vi "Test Case Result Skipped Count.vi"(8 "error in (no error)":errorcluster, 11 "Test Test Case Result In":refnum<class "Test Case Result Test.lvclass">) -> (0 "error out":errorcluster, 3 "Test Test Case Result Out":refnum<class "Test Case Result Test.lvclass">)   [LabVIEW 2020, in "LUnit Tests.lvlib" / "Test Case Result Test.lvclass"]
uses:
  Test Case Result Test.lvclass
  C:/Program Files (x86)/National Instruments/LabVIEW 2020/vi.lib/Asteme/LUnit/Test Case.lvclass
  Test Dummys/Test Test Case/Test Test Case.lvclass
  C:/Users/anton/Documents/GitHub/LUnit/source/Framework/Test Case/LUnit Test Case.lvclass
  source/Framework/Result Classes/Test Case Result/Test Case Result.lvclass/Test Case Result.ctl
  source/Framework/Result Classes/Method Result/Method Result.lvclass/Method Result.ctl
  <vilib>/Asteme/LUnit/Test Case.lvclass/Test Case.ctl
  <vilib>/Asteme/LUnit/LUnit Assertion Result.lvclass/LUnit Assertion Result.ctl
  <vilib>/Asteme/LUnit/LUnit Test Case Result.lvclass/LUnit Test Case Result.ctl
  <vilib>/Asteme/LUnit/LUnit Method Result.lvclass/LUnit Method Result.ctl
  source/Framework/Result Classes/Test Case Result/Private/SubVIs/Count by Status.vi
  <vilib>/Asteme/LUnit/Palette/Pass.vi
  <vilib>/Asteme/LUnit/Palette/Fail.vi
  <vilib>/Asteme/LUnit/Variant to string.vi
  <vilib>/Asteme/LUnit/Set Assertion Type.vi
  source/Framework/Result Classes/Method Result/Public/Read Status.vi
  <vilib>/Asteme/LUnit/Add test result.vi
  <vilib>/Asteme/LUnit/LUnit Write Passed.vi
  <vilib>/Asteme/LUnit/LUnit Write Message.vi
  <vilib>/Asteme/LUnit/LUnit Write Description.vi
  <vilib>/Asteme/LUnit/LUnit Write Assertion Type.vi
  <vilib>/Asteme/LUnit/LUnit Record Assertion Result.vi
  <vilib>/Asteme/LUnit/LUnit Aggregate Assertion Results.vi
  <vilib>/Asteme/LUnit/Assertion Result/LUnit Read Status.vi
  <vilib>/Asteme/LUnit/LUnit Read Message.vi
  <vilib>/Asteme/LUnit/LUnit Read Description.vi
  <vilib>/Asteme/LUnit/Method Result/LUnit Merge Status.vi
  <vilib>/Asteme/LUnit/LUnit Concatenate result strings.vi
  <vilib>/Utility/Data Type/Get Type Information.vi
  <vilib>/Utility/LVClass/Get LV Class Name.vi
  <vilib>/Asteme/LUnit/LUnit Assertion Result.lvclass
  source/Framework/Result Classes/Test Case Result/Test Case Result.lvclass
  <vilib>/Asteme/LUnit/Test Case.lvclass
  C:/Users/anton/Documents/GitHub/LUnit/tests/Test Dummys/Test Test Case/Test Test Case.lvclass
  C:/Users/anton/Documents/GitHub/LUnit/tests/Framework Test/Test Test Case Result/Test Case Result Test.lvclass
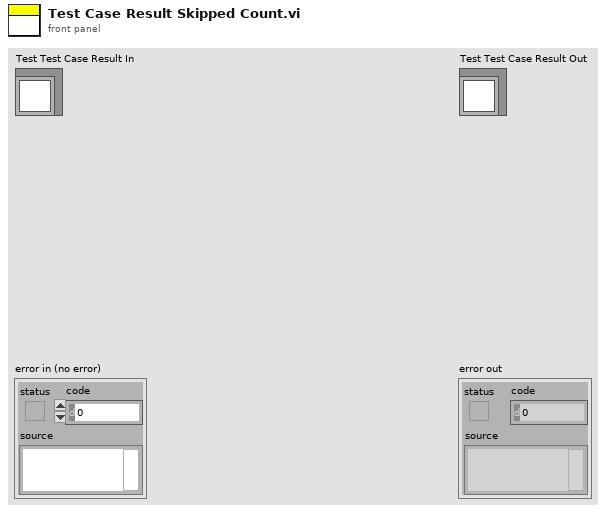
[diagram p1: front panel]
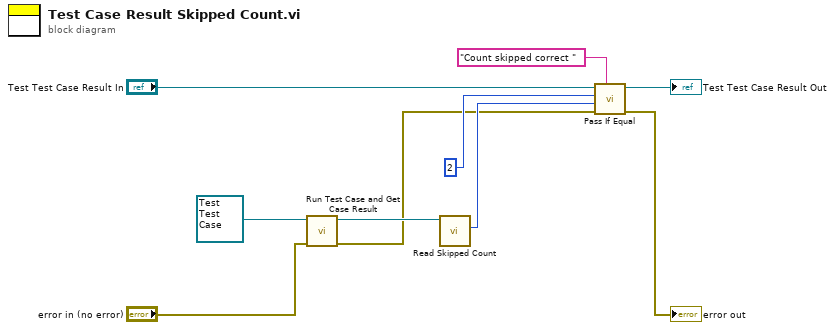
[diagram p0: block diagram]
diagram:
  n1 = call "Run Test Case and Get Case Result.vi"("error in (no error)"="error in (no error)", "Error First Test Case in"=refnum<class "Test Test Case.lvclass"> refnum ("Test Test Case.lvclass")) -> ("error out"=w3:errorcluster, "Test Case Result out"=w4:refnum<class "Test Case Result.lvclass">)  [unwired: 8 in]
  n2 = call "Read Skipped Count.vi"("Test Case Result In"=w4) -> ("Skipped count"=w5:i32)  [unwired: 9 in, 1 out]
  n3 = call <vilib>:"Pass If Equal.vi"("Description"="Count skipped correct ", "error in (no error)"=w3, "Actual"=w5, "Expected"=2 ("x"), "LUnit Test Case In"="Test Test Case Result In") -> ("error out"=→"error out":errorcluster, "LUnit Test Case Out"=→"Test Test Case Result Out":refnum<class "Test Case Result Test.lvclass">)  [unwired: 5 in]
